vi "AODO-Synchronize Tasks.vi"(0 "Tasks In":T1[](array[typedef]), 7 "external trig":bool, 9 "Trig Src":string, 11 "error in (no error)":errorcluster) -> (4 "Tasks Out":T1[](array[typedef]), 8 "Sync Task":refnum<k21>, 10 "Start Trigger Terminal":string, 15 "error out":errorcluster)   [LabVIEW 2020]
uses:
  Typedefs/AODO-Task Specification.ctl
  <vilib>/DAQmx/configure/trigger.llb/DAQmx Start Trigger (Digital Edge).vi
  <resource>/objmgr/daqmx.rc
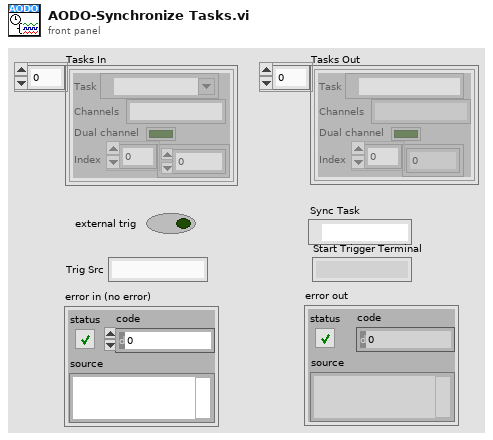
[diagram p1: front panel]
types:
  T1 = typedef "AODO-Task Specification.ctl" = cluster{"Task":refnum<k21>, "Channels":string, "Dual channel":bool, "Index":i32[]}
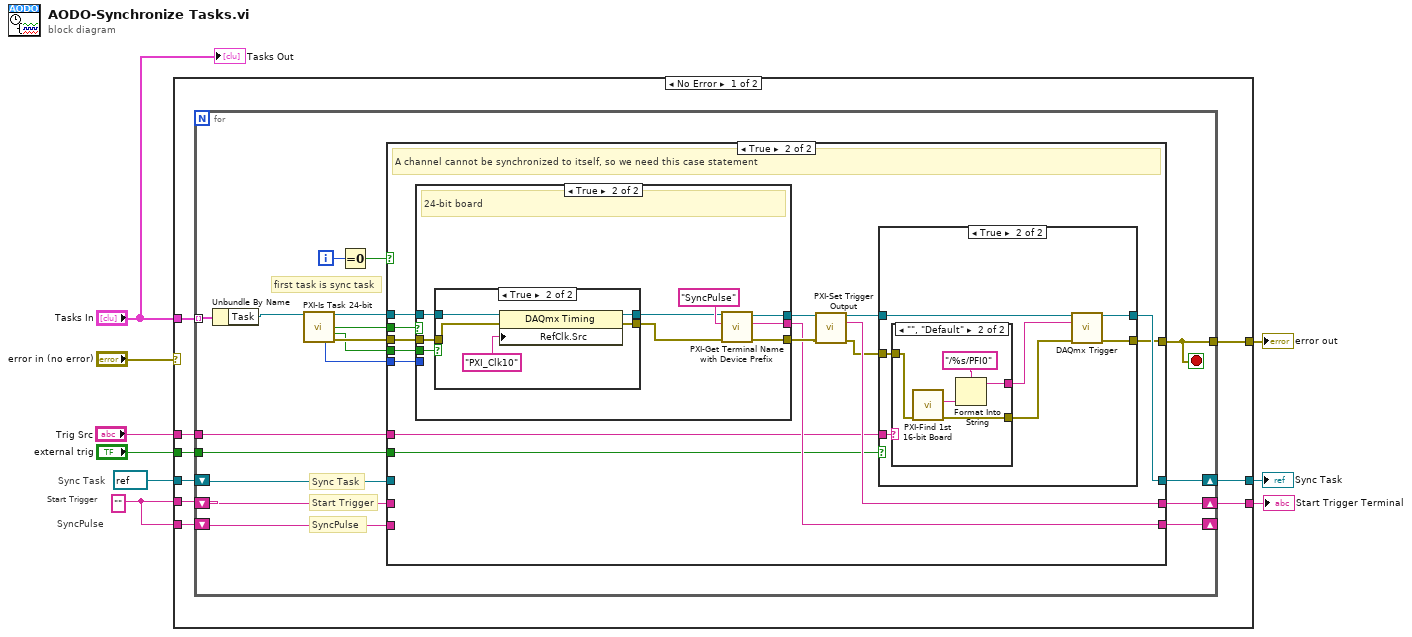
[diagram p0: block diagram]
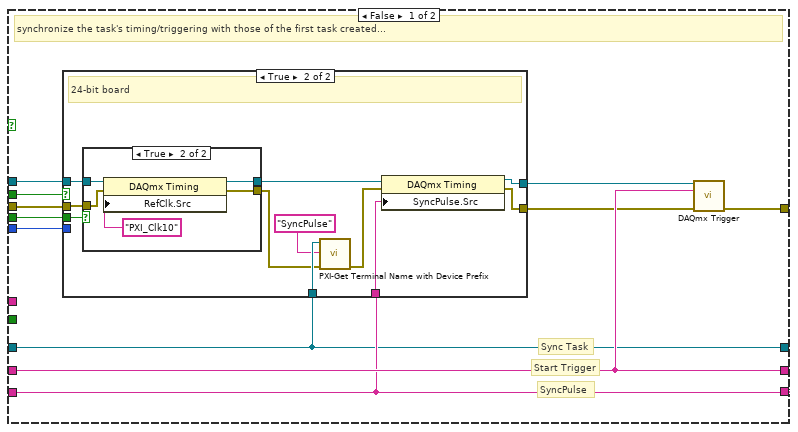
[diagram p2: hidden frame]
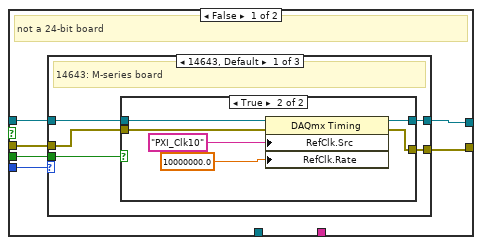
[diagram p3: hidden frame]
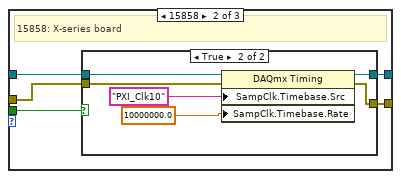
[diagram p5: hidden frame]
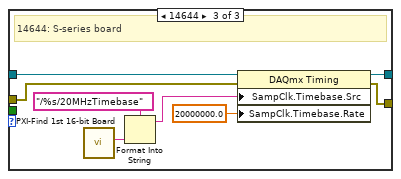
[diagram p7: hidden frame]
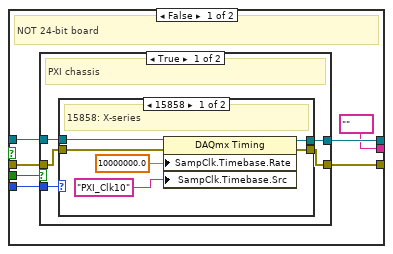
[diagram p11: hidden frame]
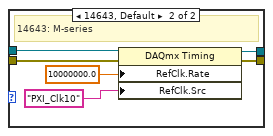
[diagram p12: hidden frame]
diagram:
  w2 = ""
  # "SyncPulse"
  # "Start Trigger"
  # "Sync Task"
  n1 = case shown="No Error" "error in (no error)" {
    selector: "error in (no error)" -> [_ w179]
    tunnel: refnum<k21> refnum ("task out") -> [w18 _]
    tunnel: w2 -> [w17 _]
    tunnel: w2 -> [w16 _]
    tunnel: "Tasks In" -> [w15 _]
    tunnel: [w14 w179] -> w6
    tunnel: [w13 _] -> w5
    tunnel: "external trig" -> [w12 _]
    tunnel: "Trig Src" -> [w11 _]
    tunnel: [w10 _] -> w1
    frame No Error {
      n2 = for {
        shift-right: [w36] -> w13
        shift-left: w18 -> [w24]
        shift-right: [w34] -> w10
        shift-left: w17 -> [w23]
        shift-right: [w33] -> _
        shift-left: w16 -> [w22]
        tunnel: [w28] -> w14
        tunnel: w15 -> [w26] mode=indexing
        tunnel: w12 -> [w21]
        tunnel: w11 -> [w20]
        i -> [w35]
        stop <- w28 stop-if-true
        # "SyncPulse"
        # "Start Trigger"
        # "Sync Task"
        # "first task is sync task"
        n3 = Unbundle By Name(w26) -> ("Task"=w25:refnum<k21>)
        n4 = call "PXI-Is Task 24-bit.vi"("task"=w25) -> ("task out"=w30:refnum<k21>, "is 24bit?"=w27:bool, "PXI?"=w19:bool, "Product Category"=w29:i32, "error out"=w31:errorcluster)  [unwired: 9 in, 1 out]
        n5 = Equal To 0?(x=w35) -> (x = 0?=w32:bool)
        n6 = case shown="True" w32 {
          tunnel: w31 -> [w45 w115]
          tunnel: [w47 w108] -> w28
          tunnel: [w39 w109] -> w36
          tunnel: w24 -> [w39 _]
          tunnel: [w46 w117] -> w34
          tunnel: w23 -> [w46 _]
          tunnel: [w44 w118] -> w33
          tunnel: w22 -> [w44 _]
          tunnel: w30 -> [w40 w116]
          tunnel: w27 -> [w41 w114]
          tunnel: w29 -> [w38 w113]
          tunnel: w19 -> [w37 w112]
          tunnel: w21 -> [_ w107]
          tunnel: w20 -> [_ w106]
          frame False {
            # "SyncPulse"
            # "Start Trigger"
            # "Sync Task"
            # "synchronize the task's timing/triggering with those of the first task created..."
            n7 = case shown="True" w41 {
              tunnel: [w51 w98] -> w43
              tunnel: [w52 w97] -> w42
              tunnel: w39 -> [_ w96]
              tunnel: w45 -> [w49 w95]
              tunnel: w44 -> [_ w94]
              tunnel: w40 -> [w50 w89]
              tunnel: w38 -> [w53 _]
              tunnel: w37 -> [w48 w88]
              frame False {
                # "not a 24-bit board"
                n8 = case shown="14643, Default" w53 {
                  tunnel: [w58 w71 w87] -> w51
                  tunnel: [w57 w70 w86] -> w52
                  tunnel: w50 -> [w56 w69 w84]
                  tunnel: w49 -> [w55 w68 w83]
                  tunnel: w48 -> [w54 w67 _]
                  frame 14643, Default {
                    # "14643: M-series board"
                    n9 = case shown="True" w54 {
                      tunnel: [w60 w66] -> w58
                      tunnel: [w59 w65] -> w57
                      tunnel: w56 -> [w60 w62]
                      tunnel: w55 -> [w59 w61]
                      frame False {
                      }
                      frame True {
                        n10 = property class="DAQmx Timing"(reference=w62, error in=w61, "RefClk.Src"="PXI_Clk10", "RefClk.Rate"=10000000.0) -> (reference out=w66:refnum<k21>, error out=w65:errorcluster)
                      }
                    }
                  }
                  frame 15858 {
                    # "15858: X-series board"
                    n11 = case shown="True" w67 {
                      tunnel: [w73 w79] -> w71
                      tunnel: [w72 w78] -> w70
                      tunnel: w69 -> [w73 w75]
                      tunnel: w68 -> [w72 w74]
                      frame False {
                      }
                      frame True {
                        n12 = property class="DAQmx Timing"(reference=w75, error in=w74, "SampClk.Timebase.Src"="PXI_Clk10" ("RefClk.Src"), "SampClk.Timebase.Rate"=10000000.0) -> (reference out=w79:refnum<k21>, error out=w78:errorcluster)
                      }
                    }
                  }
                  frame 14644 {
                    # "14644: S-series board"
                    n13 = call "PXI-Find 1st 16-bit Board.vi"() -> ("DAQmx Device Name"=w80:tag)  [unwired: 9 in, 2 out]
                    n14 = Format Into String(format string="/%s/20MHzTimebase", w80) -> (resulting string=w81:string)  [unwired: 2 in, 1 out]
                    n15 = property class="DAQmx Timing"(reference=w84, error in=w83, "SampClk.Timebase.Src"=w81, "SampClk.Timebase.Rate"=20000000.0) -> (reference out=w87:refnum<k21>, error out=w86:errorcluster)
                  }
                }
              }
              frame True {
                # "24-bit board"
                n16 = case shown="True" w88 {
                  tunnel: w95 -> [w99 w105]
                  tunnel: [w99 w104] -> w91
                  tunnel: [w100 w103] -> w90
                  tunnel: w89 -> [w100 w102]
                  frame False {
                  }
                  frame True {
                    n17 = property class="DAQmx Timing"(reference=w102, error in=w105, "RefClk.Src"="PXI_Clk10") -> (reference out=w103:refnum<k21>, error out=w104:errorcluster)
                  }
                }
                n18 = call "PXI-Get Terminal Name with Device Prefix.vi"("error in (no error)"=w91, "Local Terminal Name"="SyncPulse", "task/channels in"=w96) -> ("error out"=w92:errorcluster)  [unwired: 6 in, 2 out]
                n19 = property class="DAQmx Timing"(reference=w90, error in=w92, "SyncPulse.Src"=w94) -> (reference out=w98:refnum<k21>, error out=w97:errorcluster)
              }
            }
            n20 = call-poly <vilib>:"DAQmx Trigger.vi"("task/channels in"=w43, "source"=w46, "error in"=w42) -> ("error out"=w47:errorcluster)  [unwired: 11 in, 1 out]
          }
          frame True {
            # "A channel cannot be synchronized to itself, so we need this case statement"
            n21 = case shown="True" w114 {
              tunnel: [w142 w171] -> w119
              tunnel: w116 -> [w143 w165]
              tunnel: [w141 w170] -> w120
              tunnel: w115 -> [w140 w164]
              tunnel: [tag "" ("Terminal Name with Device Prefix") w169] -> w118
              tunnel: w113 -> [w137 _]
              tunnel: w112 -> [w138 w163]
              frame False {
                # "NOT 24-bit board"
                n22 = case shown="True" w138 {
                  tunnel: w143 -> [w148 w162]
                  tunnel: [w147 w162] -> w142
                  tunnel: [w146 w161] -> w141
                  tunnel: w140 -> [w145 w161]
                  tunnel: w137 -> [w144 _]
                  frame True {
                    # "PXI chassis"
                    n23 = case shown="15858" w144 {
                      tunnel: w148 -> [w154 w160]
                      tunnel: [w153 w159] -> w147
                      tunnel: [w152 w158] -> w146
                      tunnel: w145 -> [w151 w157]
                      frame 15858 {
                        # "15858: X-series"
                        n24 = property class="DAQmx Timing"(reference=w154, error in=w151, "SampClk.Timebase.Rate"=10000000.0, "SampClk.Timebase.Src"="PXI_Clk10" ("RefClk.Src")) -> (reference out=w153:refnum<k21>, error out=w152:errorcluster)
                      }
                      frame 14643, Default {
                        # "14643: M-series"
                        n25 = property class="DAQmx Timing"(reference=w160, error in=w157, "RefClk.Rate"=10000000.0, "RefClk.Src"="PXI_Clk10") -> (reference out=w159:refnum<k21>, error out=w158:errorcluster)
                      }
                    }
                  }
                  frame False {
                    # "NOT PXI chassis"
                  }
                }
              }
              frame True {
                # "24-bit board"
                n26 = case shown="True" w163 {
                  tunnel: [w173 w178] -> w167
                  tunnel: [w172 w177] -> w166
                  tunnel: w165 -> [w173 w176]
                  tunnel: w164 -> [w172 w175]
                  frame False {
                  }
                  frame True {
                    n27 = property class="DAQmx Timing"(reference=w176, error in=w175, "RefClk.Src"="PXI_Clk10") -> (reference out=w178:refnum<k21>, error out=w177:errorcluster)
                  }
                }
                n28 = call "PXI-Get Terminal Name with Device Prefix.vi"("error in (no error)"=w166, "Local Terminal Name"="SyncPulse", "task/channels in"=w167) -> ("error out"=w170:errorcluster, "Terminal Name with Device Prefix"=w169:string, "task out"=w171:refnum<k21>)  [unwired: 6 in]
              }
            }
            n29 = call "PXI-Set Trigger Output.vi"("Task in"=w119, "error in (no error)"=w120) -> ("Task out"=w110:refnum<k21>, "Trigger Terminal"=w117:string, "error out"=w111:errorcluster)  [unwired: 11 in]
            n30 = case shown="True" w107 {
              tunnel: [w121 w129] -> w108
              tunnel: w110 -> [w122 w128]
              tunnel: w111 -> [w121 w126]
              tunnel: [w122 w127] -> w109
              tunnel: w106 -> [_ w123]
              frame False {
              }
              frame True {
                n31 = case shown="\"\", \"Default\"" w123 {
                  selector: w123 -> [w131 _]
                  tunnel: w126 -> [w130 w136]
                  tunnel: [w130 w135] -> w125
                  tunnel: [w131 w132] -> w124
                  frame "else", Default {
                  }
                  frame "", "Default" {
                    n32 = call "PXI-Find 1st 16-bit Board.vi"("error in (no error)"=w136) -> ("error out"=w135:errorcluster, "DAQmx Device Name"=w134:tag)  [unwired: 8 in, 1 out]
                    n33 = Format Into String(format string="/%s/PFI0", w134) -> (resulting string=w132:string)  [unwired: 2 in, 1 out]
                  }
                }
                n34 = call-poly <vilib>:"DAQmx Trigger.vi"("task/channels in"=w128, "source"=w124, "error in"=w125) -> ("task out"=w127:refnum<k21>, "error out"=w129:errorcluster)  [unwired: 11 in]
              }
            }
          }
        }
      }
    }
    frame Error {
    }
  }
  "error out" <- w6
  "Sync Task" <- w5
  "Start Trigger Terminal" <- w1
  "Tasks Out" <- "Tasks In"
